vi "Int64 Create.vi"(8 "error in (no error)":errorcluster, 11 "I64 in":i64) -> (0 "error out":errorcluster, 3 "Int64 DVR out":refnum<data-value>)   [LabVIEW 2012, in "MDSplus.lvlib"]
uses:
  <vilib>/MDSplus/Library/MDSplus.lvlib
  <vilib>/MDSplus/Classes/Data_Class/Scalar_Class/Int64_Class/Int64.lvclass
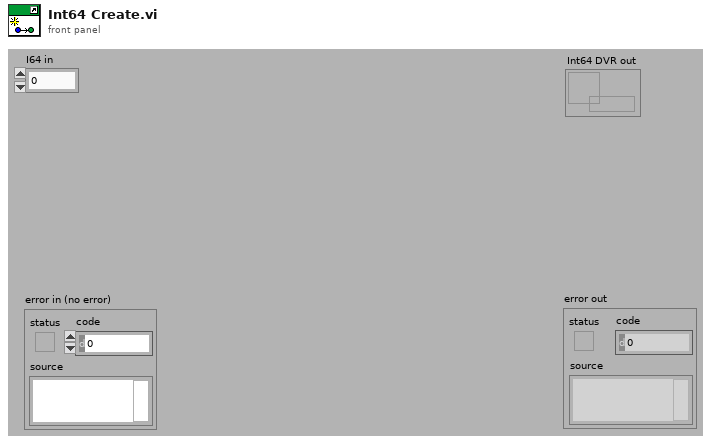
[diagram p1: front panel]
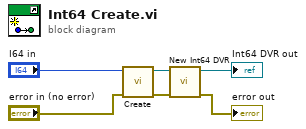
[diagram p0: block diagram]
diagram:
  n1 = call <vilib>:"Create.vi"("error in (no error)"="error in (no error)", "I64 in"="I64 in") -> ("error out"=w3:errorcluster, "Int64 out"=w4:refnum<class "Int64.lvclass">)  [unwired: 8 in]
  n2 = call <vilib>:"New Int64 DVR.vi"("error in (no error)"=w3, "Int64 in"=w4) -> ("error out"=→"error out":errorcluster, "Int64 DVR out"=→"Int64 DVR out":refnum<data-value>)  [unwired: 8 in]
